vi "Database.Handler.Connect.vi"(6 "ReInitDLL (F)":bool, 8 "error in":errorcluster, 11 "Data in":T1) -> (0 "error out":errorcluster, 3 "Data out":T1)   [LabVIEW 2016]
doc: "Connect to database\n\nWabco 2017 All right reserved\nAuthor: maciej.szupienko@wabco-auto.com"
uses:
  Database.Handler.Data.ctl
  Database.Handler.Data.Status.ctl
  Database.Handler.Data.Sets.ctl
  Tools/Translator/Translator.Message.ctl
  Tools/EventLog/EventLog.EventSource.ctl
  Tools/EventLog/EventLog.New(array).vi
  Tools/EventLog/EventLog.CreateError(array).vi
  Tools/ErrorHandling/ErrorHandling.Create.vi
  Global/ApplicationGlobal.vi
  Tools/EventLog/EventLog.Buffer.vi
  Tools/EventLog/EventLog.File.ReadWrite.vi
  Tools/Tma.lib/string.llb/Join array to string.vi
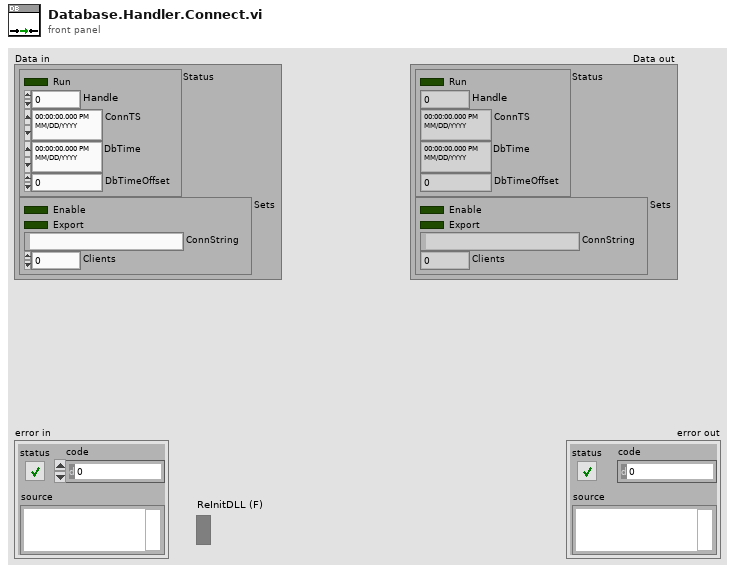
[diagram p1: front panel]
types:
  T1 = typedef "Database.Handler.Data.ctl" = cluster{"Status":T2, "Sets":T3}
  T2 = typedef "Database.Handler.Data.Status.ctl" = cluster{"Run":bool, "Handle":i32, "ConnTS":timestamp, "DbTime":timestamp, "DbTimeOffset":dbl}
  T3 = typedef "Database.Handler.Data.Sets.ctl" = cluster{"Enable":bool, "Export":bool, "ConnString":string, "Clients":i32}
  T4 = typedef "Translator.Message.ctl" = enum16{"-", "Event confirmed", "Log out", "Log in", "Shutdown", "Cancel", "Start", "Continue", "Stop", "On", "Off", "OK", "NOK", "NOK %s", "This", "Prev", "Home", "Work", "In progress...", "Missing", "Empty", "Hardware failure", "Initial", "Error %d >> %s", "Error %d >> %s >> %s", "Starting %s", "Quitting %s", "Configured", "Initializing", "Quitting", "Loading", "Running %s", "Stopped", "Summary", "Do you want to continue?", "Do you want to exit?", "Log out?", "System", "All", "IDLE", "Translating...%s", "Not found", "Alarm %s", "Run", "Skip", "Abort", "Repeat", "Please wait...", "Database disconnected", "Login to database successful", "Login to database failed: %d; %s", "Get process step data for %s", "Changeover off", "Changeover into %s", "Product %s | %s found in cache with status %d at previous station", "Product %s | %s found in database with status %d at previous station", "Product %s | %s not found in cache at previous station", "Product %s | %s not found in database at previous station", "Product %s | %s found in cache with status %d at this station (%d repetion)", "Product %s | %s found in database with status %d at this station (%d repetition)", "Product %s | %s not found in cache at this station", "Product %s | %s not found in database at this station", "Product %s | %s found in cache for component %s | %s", "Product %s | %s found in database for component %s | %s", "Product not found in cache for component %s | %s", "Product not found in database for component %s | %s", "Product %s | %s connected with component %s | %s (cache)", "Product %s | %s connected with component %s | %s (database)", "New data for %s | %s (cache)", "New data for %s | %s (database)", "File %s moved (cache)", "File %s deleted (cache)", "Msg %d >> %s", "PLC LifeBit Failure", "Reconnecting DB", "Reconnecting PLC", "Free disk space is below 1GB - contact technician"}
  T5 = typedef "EventLog.EventSource.ctl" = enum16{"All", "Gui", "Cache", "PLC1", "PLC2", "PLC3", "DB", "DB01", "DB02", "DB03", "DB04", "DB05", "DB06", "DB07", "DB08", "DB09", "DB10", "DB11", "DB12", "DB13", "DB14", "DB15", "DB16"}
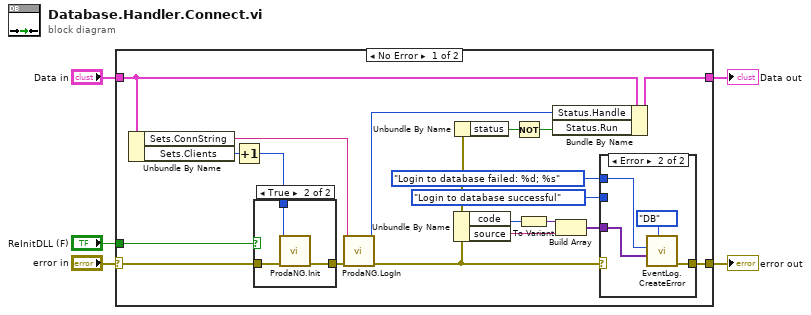
[diagram p0: block diagram]
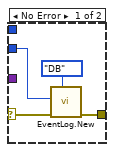
[diagram p3: hidden frame]
diagram:
  n1 = case shown="No Error" "error in" {
    selector: "error in" -> [w10 w38]
    tunnel: [w17 w38] -> w5
    tunnel: [w22 w37] -> w4
    tunnel: "Data in" -> [w21 w37]
    tunnel: "ReInitDLL (F)" -> [w8 _]
    frame No Error {
      n2 = Unbundle By Name(w21) -> ("Sets.ConnString"=w11:string, "Sets.Clients"=w7:i32)
      n3 = Increment(x=w7) -> (x+1=w6:i32)
      n4 = case shown="True" w8 {
        tunnel: w10 -> [w25 w28]
        tunnel: [w25 w27] -> w9
        tunnel: w6 -> [_ w26]
        frame False {
        }
        frame True {
          n5 = call "ProdaNG.Init.vi"("error in (no error)"=w28, "numContexts (0: unlimited)"=w26) -> ("error out"=w27:errorcluster)  [unwired: 9 in]
        }
      }
      n6 = call "ProdaNG.LogIn.vi"("error in"=w9, "ConnectionString"=w11) -> ("error out"=w16:errorcluster, "dbHandle"=w12:i32)  [unwired: 7 in, 1 out]
      n7 = Unbundle By Name(w16) -> ("code"=w20:i32, "source"=w18:string)
      n8 = Unbundle By Name(w16) -> ("status"=w23:bool)
      n9 = Not(x=w23) -> (.not. x?=w24:bool)
      n10 = To Variant(anything=w20) -> (Variant=w19:variant)
      n11 = Bundle By Name(cluster=w21, "Status.Handle"=w12, "Status.Run"=w24) -> (w22:T1)
      n12 = Build Array(w19, w18) -> (w15:variant[])
      n13 = case shown="Error" w16 {
        selector: w16 -> [w30 _]
        tunnel: [w32 w36] -> w17
        tunnel: w15 -> [_ w35]
        tunnel: Translator.Message."Login to database failed: %d; %s" ("Message (-)") -> [_ w34]
        tunnel: Translator.Message."Login to database successful" ("Message (-)") -> [w31 _]
        frame No Error {
          n14 = call-poly "EventLog.New.vi"("Source (All)"=EventLog.EventSource."DB", "error in (no error)"=w30, "Message (-)"=w31) -> ("error out"=w32:errorcluster)  [unwired: 7 in, 1 out]
        }
        frame Error {
          n15 = call-poly "EventLog.CreateError.vi"("Source (All)"=EventLog.EventSource."DB", "args"=w35, "Msg"=w34) -> ("error out"=w36:errorcluster)  [unwired: 7 in, 1 out]
        }
      }
    }
    frame Error {
    }
  }
  "error out" <- w5
  "Data out" <- w4
